vi "Read N Records.vi"(7 "Timeout (s)":dbl=10.0, 8 "error in":errorcluster, 11 "FPGA VI Reference In":refnum<k20>) -> (0 "error out":errorcluster, 1 "Channel 1 Records":i16[][](array[numeric]), 2 "Channel 0 Records":i16[][](array[numeric]), 3 "FPGA VI Reference Out":refnum<k20>, 4 "Elements Remaining":u32, 6 "Records Done":u32)   [LabVIEW 2011]
panel:
  out "Num U64s":u32
  out "Records to Acquire":u32
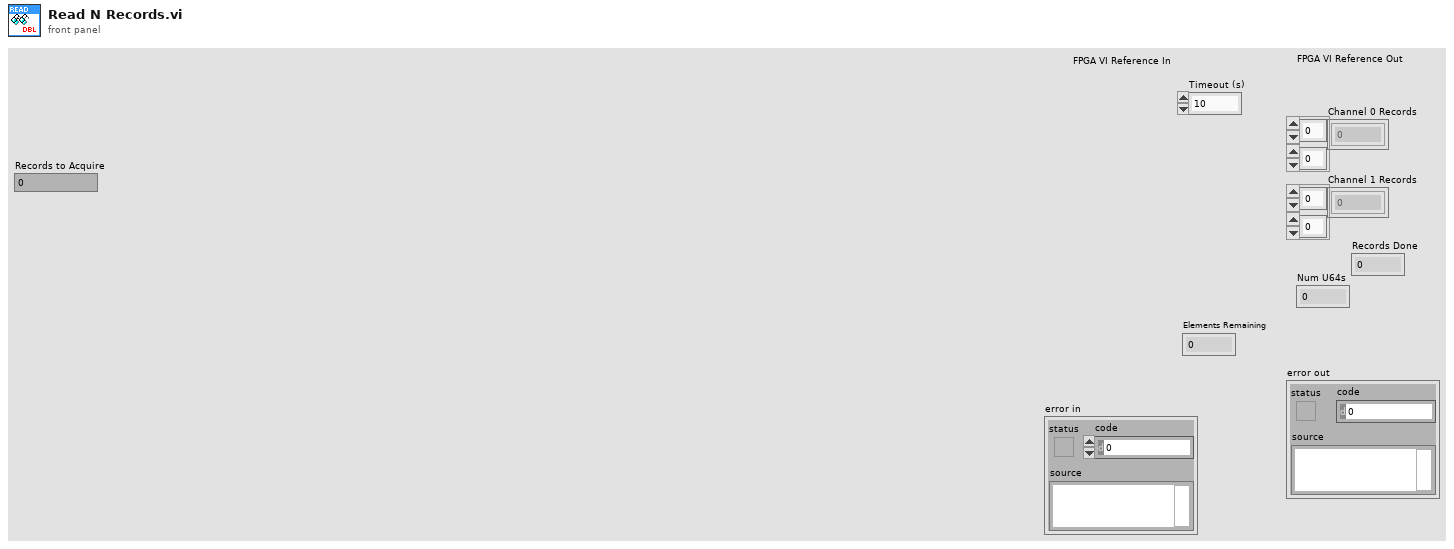
[diagram p1: front panel]
types:
  T1 = cluster{"DRAM Write Ticks":u16, "DRAM Read Ticks":u16}
  T2 = cluster{"write grant time (clocks)":u16, "read grant time (clocks)":u16}
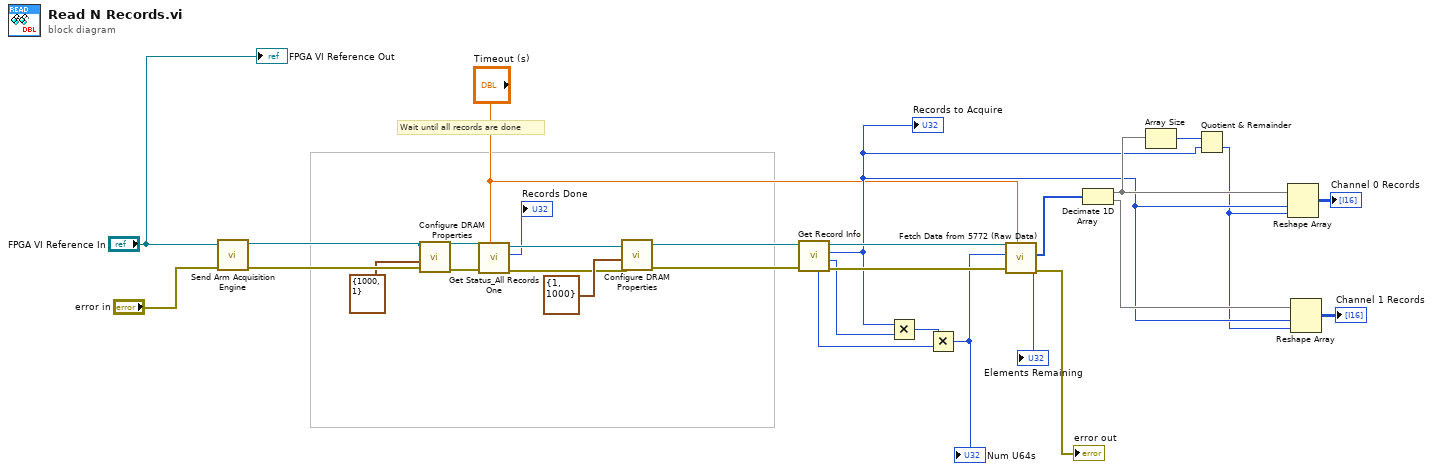
[diagram p0: block diagram]
diagram:
  # "Wait until all records are done"
  n1 = call <userlib>:"Send Arm Acquisition Engine.vi"("error in"="error in", "FPGA VI Reference In"="FPGA VI Reference In") -> ("error out"=w29:errorcluster, "FPGA VI Reference Out"=w30:refnum<k20>)  [unwired: 8 in]
  n2 = call <userlib>:"Configure DRAM Properties.vi"("error in"=w29, "DRAM Duty Cycle"=T2 {"write grant time (clocks)"=1000, "read grant time (clocks)"=1} ("DRAM Arbiter Config"), "FPGA VI Reference In"=w30) -> ("error out"=w25:errorcluster, "FPGA VI Reference Out"=w26:refnum<k20>)  [unwired: 7 in]
  n3 = call <userlib>:"Get Status_All Records One.vi"("Timeout (s)"="Timeout (s)", "error in"=w25, "FPGA VI Reference In"=w26) -> ("error out"=w24:errorcluster, "Records Done"=→"Records Done":u32, "FPGA VI Reference Out"=w23:refnum<k20>)  [unwired: 6 in]
  n4 = call <userlib>:"Configure DRAM Properties.vi"("error in"=w24, "DRAM Duty Cycle"=T1 {"DRAM Write Ticks"=1, "DRAM Read Ticks"=1000}, "FPGA VI Reference In"=w23) -> ("error out"=w21:errorcluster, "FPGA VI Reference Out"=w22:refnum<k20>)  [unwired: 7 in]
  n5 = call <userlib>:"Get Record Info.vi"("error in"=w21, "FPGA VI Reference In"=w22) -> ("error out"=w20:errorcluster, "Record Length"=w12:u32, "Records to Acquire"=w14:u32, "FPGA VI Reference Out"=w19:refnum<k20>, "Num of Channels"=w5:u32)  [unwired: 5 in]
  "Records to Acquire" <- w14
  n6 = Multiply(x=w14, y=w12) -> (x*y=w6:u32)
  n7 = Multiply(x=w6, y=w5) -> (x*y=w4:u32)
  "Num U64s" <- w4
  n8 = call <userlib>:"Fetch Data from 5772 (Raw Data).vi"("Timeout (s)"="Timeout (s)", "error in"=w20, "Samples"=w4, "FPGA VI Reference In"=w19) -> ("error out"=→"error out":errorcluster, "Data Acquired"=w17:i16[], "Elements Remaining"=→"Elements Remaining":u32)  [unwired: 4 in, 1 out]
  n9 = Decimate 1D Array(w17) -> (w16:i16[], w18:i16[])
  n10 = Array Size(array=w16) -> (size(s)=w15:i32)
  n11 = Quotient & Remainder(x=w15, y=w14) -> (floor(x/y)=w13:u32)  [unwired: 1 out]
  n12 = Reshape Array(w16, w14, w13) -> (→"Channel 0 Records":i16[][])
  n13 = Reshape Array(w18, w14, w13) -> (→"Channel 1 Records":i16[][])
  "FPGA VI Reference Out" <- "FPGA VI Reference In"
